vi "Write XML Handler.lvclass.vi"(10 "XML Handler.lvclass":refnum<class "XML Handler.lvclass">, 11 "Test Framework in":refnum<class "Test Framework.lvclass">) -> (3 "Test Framework out":refnum<class "Test Framework.lvclass">)   [LabVIEW 2020, in "Test Framework.lvclass"]
uses:
  Test Framework.lvclass
  XML Handler/XML Handler.lvclass
  Test Framework.lvclass/Test Framework.ctl
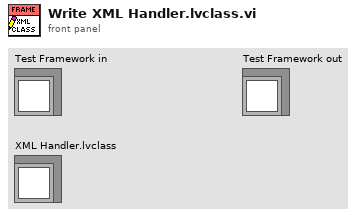
[diagram p1: front panel]
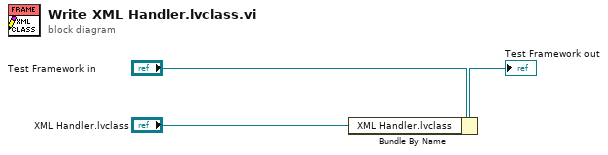
[diagram p0: block diagram]
diagram:
  n1 = Bundle By Name(cluster="Test Framework in", "XML Handler.lvclass"="XML Handler.lvclass") -> (→"Test Framework out":refnum<class "Test Framework.lvclass">)
